vi "array-normalization.vi"(1 "Array":dbl[][](array[numeric])) -> (0 "x/y":dbl[][](array[numeric]))   [LabVIEW 2021]
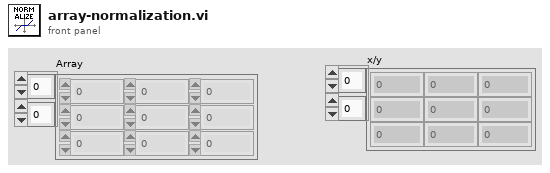
[diagram p1: front panel]
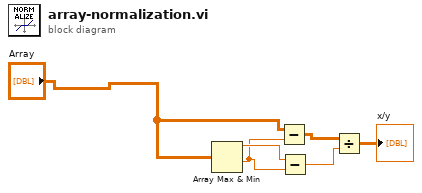
[diagram p0: block diagram]
diagram:
  n1 = Array Max & Min(array="Array") -> (max value=w6:dbl, min value=w5:dbl)  [unwired: 2 out]
  n2 = Subtract(x="Array", y=w5) -> (x-y=w4:dbl[][])
  n3 = Subtract(x=w6, y=w5) -> (x-y=w3:dbl)
  n4 = Divide(x=w4, y=w3) -> (x/y=→"x/y":dbl[][])
